vi "agilent_monitor.vi"(6 "Thermal Coefficient Path":path, 7 "Action":u8(ring) items=["initialize", "read new values", "read last values"], 8 "Temperature Readings":u16=1, 9 "Voltage Readings":u16=3, 10 "voltage channels (csv)":string, 11 "Agilent Port In":refnum<visa-resource-name>="COM35") -> (0 "voltage stdvs":dbl[](array[numeric]) format="%.6f", 1 "voltages":dbl[](array[numeric]), 2 "TempProbeSet out":refnum<class "TempProbeSet.lvclass">)   [LabVIEW 2010]
doc: "This VI is an Action Engine (see the community nugget by Ben on the labview forums - a quick google for \"action engine labview\" will do)\n\nIn order to use it, you must first call it with \"initialize\" passed as the first action while also specifying the agilent port, the path to the thermal coefficients file, and a string with voltage channel numbers separated by commas. These values will be stored for subsequent querries for data.\n\nTo query for data, just pass in the number of voltage readings and temperature readings desired\n\nAt the moment, getting the temperature data out of this beast required using the probe_temps.vi on the TempProbeSet out terminal. This takes an array of location names (as found in the thermal coefficients file) and spits out the corresponding array of temps.\n\nGetting voltage is more straightforward - simply take the voltage readings array from this beast and do what ye will with it."
uses:
  ProbeClass/TempProbeSet.lvclass
panel:
  out "error out":errorcluster
  # "This VI is an Action Engine (see the community nugget by Ben on the labview forums - a quick google for \"action engine labview\" will do)\n\nIn order to use it, you must first call it with \"initialize\" passed as the first action while also specifying the agilent port, the path to the thermal coefficients file, and a string with voltage channel numbers separated by commas. These values will be stored for subsequent querries for data.\n\nTo query for data, just pass in the number of voltage readings and temperature readings desired\n\nAt the moment, getting the temperature data out of this beast required using the probe_temps.vi on the TempProbeSet out terminal. This takes an array of location names (as found in the thermal coefficients file) and spits out the corresponding array of temps.\n\nGetting voltage is more straightforward - simply take the voltage readings array from this beast and do what ye will with it."
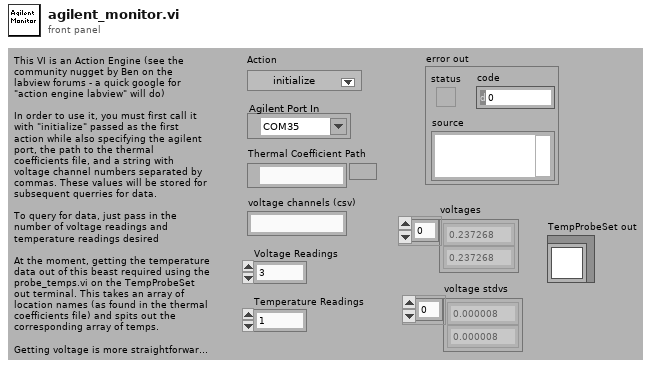
[diagram p1: front panel]
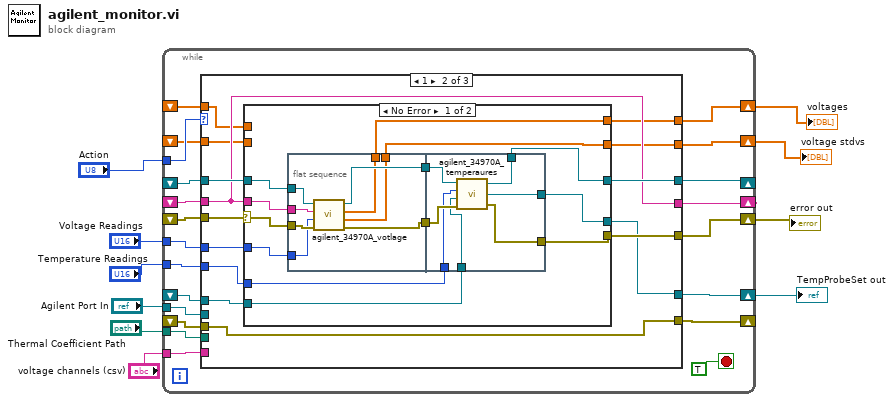
[diagram p0: block diagram]
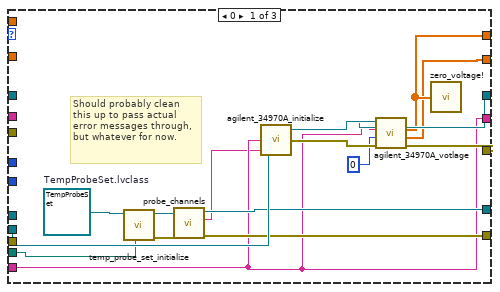
[diagram p2: hidden frame]
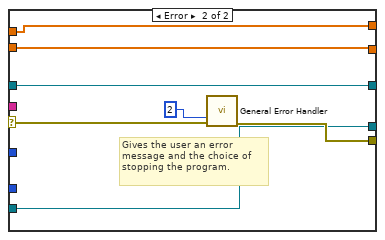
[diagram p3: hidden frame]
diagram:
  n1 = while {
    shift-right: [w30] -> _
    shift-left: _ -> [w29]
    shift-right: [w31] -> w4
    shift-left: _ -> [w26]
    shift-right: [w27] -> w3
    shift-left: _ -> [w28]
    tunnel: "Action" -> [w25]
    tunnel: "Agilent Port In" -> [w24]
    tunnel: "Thermal Coefficient Path" -> [w22]
    tunnel: "voltage channels (csv)" -> [w21]
    shift-right: [w20] -> _
    shift-left: _ -> [w19]
    tunnel: "Temperature Readings" -> [w18]
    tunnel: "Voltage Readings" -> [w17]
    shift-right: [w16] -> _
    shift-left: _ -> [w15]
    shift-right: [w13] -> w1
    shift-left: _ -> [w12]
    shift-right: [w14] -> w2
    shift-left: _ -> [w11]
    stop <- TRUE stop-if-true
    n2 = case shown="1" w25 {
      tunnel: [w44 w61 w101] -> w31
      tunnel: [w45 w60 w103] -> w30
      tunnel: w29 -> [_ w59 w103]
      tunnel: w28 -> [_ w58 w100]
      tunnel: [w38 w57 w100] -> w27
      tunnel: w26 -> [_ w56 w101]
      tunnel: w24 -> [w47 _ _]
      tunnel: w22 -> [w40 _ _]
      tunnel: w21 -> [w35 _ _]
      tunnel: [w35 w55 w102] -> w20
      tunnel: w19 -> [_ w55 w102]
      tunnel: w18 -> [_ w54 _]
      tunnel: w17 -> [_ w53 _]
      tunnel: [w36 w52 w99] -> w16
      tunnel: w15 -> [_ w52 w99]
      tunnel: [w33 w51 w97] -> w14
      tunnel: [w32 w50 w98] -> w13
      tunnel: w12 -> [_ w49 w98]
      tunnel: w11 -> [_ w48 w97]
      frame 0 {
        w41 = refnum<class "TempProbeSet.lvclass"> refnum  # TempProbeSet.lvclass
        # "Should probably clean this up to pass actual error messages through, but whatever for now."
        n3 = call "temp_probe_set_initialize.vi"("Thermal Coefficient Path"=w40, "TempProbeSet in"=w41) -> ("error out"=w37:errorcluster, "TempProbeSet out"=w39:refnum<class "TempProbeSet.lvclass">)  [unwired: 8 in]
        n4 = call "probe_channels.vi"("error in (no error)"=w37, "TempProbeSet in"=w39) -> ("error out"=w36:errorcluster, "channels"=w34:string, "TempProbeSet out"=w38:refnum<class "TempProbeSet.lvclass">)  [unwired: 6 in, 1 out]
        n5 = call "agilent_34970A_initialize.vi"("resistance channels (csv)"=w34, "voltage channels (csv)"=w35, "Agilent 34970A Port"=w47) -> ("34970A Error Out"=w43:errorcluster, "34970A Port Out"=w46:refnum<visa-resource-name>)  [unwired: 1 out]
        n6 = call "agilent_34970A_votlage.vi"("error in (no error)"=w43, "Readings"=0, "Channels"=w35, "Agilent Port In"=w46) -> ("error out"=w44:errorcluster, "Voltage Standard Deviations"=w32:dbl[], "Voltage Averages"=w33:dbl[], "Agilent Port Out"=w45:refnum<visa-resource-name>)  [unwired: 2 in]
        n7 = call "zero_voltage!.vi"("Voltages"=w33) -> ()
      }
      frame 1 {
        n8 = case shown="No Error" w56 {
          selector: w56 -> [w69 w96]
          tunnel: [w72 w95] -> w61
          tunnel: [w64 w94] -> w60
          tunnel: w59 -> [w71 w94]
          tunnel: w58 -> [w70 w93]
          tunnel: [w65 w93] -> w57
          tunnel: w55 -> [w68 _]
          tunnel: w54 -> [w67 _]
          tunnel: w53 -> [w66 _]
          tunnel: [w63 w91] -> w51
          tunnel: [w62 w90] -> w50
          tunnel: w49 -> [_ w90]
          tunnel: w48 -> [_ w91]
          frame No Error {
            n9 = flat-sequence {
              tunnel: [w82] -> w74
              tunnel: [w77] -> w73
              tunnel: w71 -> [w81]
              tunnel: w69 -> [w80]
              tunnel: w68 -> [w79]
              tunnel: w66 -> [w78]
              tunnel: [w76] -> w63
              tunnel: [w75] -> w62
              tunnel: w74 -> [w89]
              tunnel: [w87] -> w64
              tunnel: w73 -> [w86]
              tunnel: [w88] -> w72
              tunnel: w70 -> [w85]
              tunnel: w67 -> [w84]
              tunnel: [w83] -> w65
              frame #0 {
                n10 = call "agilent_34970A_votlage.vi"("error in (no error)"=w80, "Readings"=w78, "Channels"=w79, "Agilent Port In"=w81) -> ("error out"=w77:errorcluster, "Voltage Standard Deviations"=w75:dbl[], "Voltage Averages"=w76:dbl[], "Agilent Port Out"=w82:refnum<visa-resource-name>)  [unwired: 2 in]
              }
              frame #1 {
                n11 = call "agilent_34970A_temperaures.vi"("error in (no error)"=w86, "TempProbeSet in"=w85, "Readings"=w84, "Agilent Port In"=w89) -> ("error out"=w88:errorcluster, "TempProbeSet out"=w83:refnum<class "TempProbeSet.lvclass">, "Agilent Port Out"=w87:refnum<visa-resource-name>)
              }
            }
          }
          frame Error {
            # "Gives the user an error message and the choice of stopping the program."
            n12 = call <vilib>:"General Error Handler.vi"("type of dialog (OK msg:1)"=2, "error in (no error)"=w96) -> ("error out"=w95:errorcluster)  [unwired: 9 in, 4 out]
          }
        }
      }
      frame 2, Default {
      }
    }
  }
  "error out" <- w4
  "TempProbeSet out" <- w3
  "voltage stdvs" <- w1
  "voltages" <- w2
